vi "test Set Field Plot Cosmetics.vi"(8 "error in (no error)":errorcluster, 11 "TestCase in":refnum<class "FieldTests.lvclass">) -> (0 "error out":errorcluster, 3 "TestCase out":refnum<class "FieldTests.lvclass">)   [LabVIEW 2014, in "FieldTests.lvclass"]
uses:
  FieldTests.lvclass
  <vilib>/addons/_JKI Toolkits/VI Tester/TestCase.llb/TestCase.lvclass
  SPLAT/Field Class/Field.lvclass
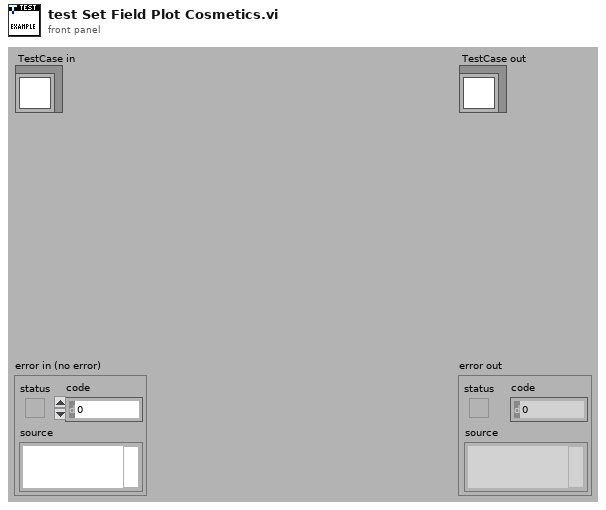
[diagram p1: front panel]
types:
  T1 = cluster{"Plot.Line Style":u8, "Plot.Line Width":u8, "Plot.Point Style":u8, "Plot.Plot Interpolation":u8, "Plot.Name":string, "Plot.Color":u32, "Fill / Point Color":u32}[]
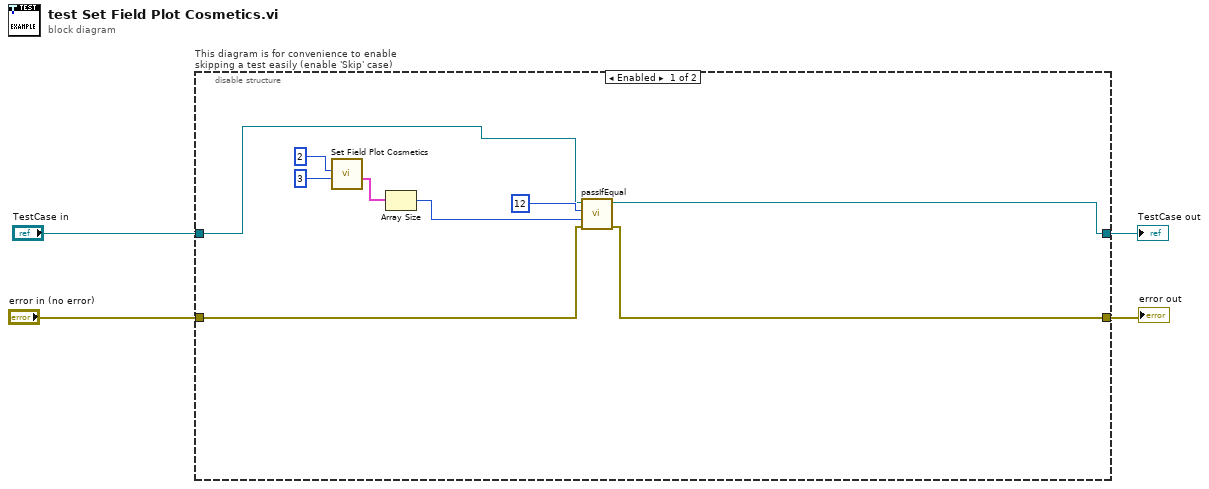
[diagram p0: block diagram]
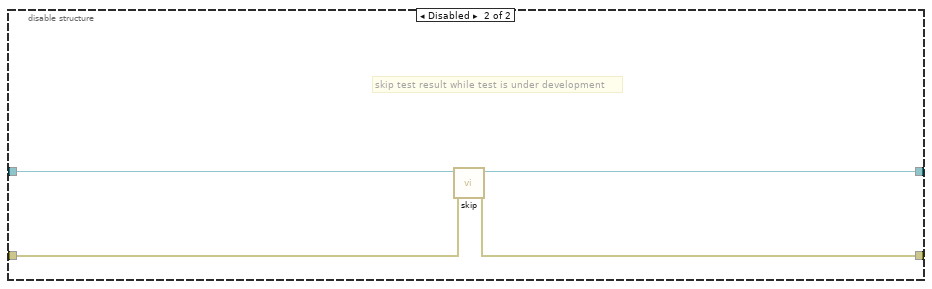
[diagram p2: hidden frame]
diagram:
  n1 = disable-structure "This diagram is for convenience to enable skipping a test easily (enable 'Skip' case)" shown="Enabled" {
    disable-tunnel: "TestCase in" -> [w8 w17]
    disable-tunnel: [w6 w15] -> w1
    disable-tunnel: [w5 w16] -> w3
    disable-tunnel: "error in (no error)" -> [w7 w14]
    frame Enabled {
      n2 = call "Set Field Plot Cosmetics.vi"("#Anchors"=3, "#Tags"=2) -> ("Field Plot Cosmetics"=w11:T1)  [unwired: 9 in]
      n3 = Array Size(array=w11) -> (size(s)=w10:i32)
      n4 = call-dynamic "passIfEqual.vi"("error in (no error)"=w7, "y"=w10, "x"=12, "TestCase in"=w8) -> ("error out"=w5:errorcluster, "TestCase out"=w6:refnum<class "FieldTests.lvclass">)  [unwired: 6 in]
    }
    frame Disabled {
      # "skip test result while test is under development"
      n5 = call <vilib>:"skip.vi"("error in (no error)"=w14, "TestCase in"=w17) -> ("error out"=w16:errorcluster, "TestCase out"=w15:refnum<class "FieldTests.lvclass">)  [unwired: 8 in]
    }
  }
  "error out" <- w3
  "TestCase out" <- w1
